vi "CalculatePositionIndex.vi"(8 "error in (no error)":errorcluster, 10 "DragPosition":i32, 11 "OrderSelection in":refnum<class "OrderSelection.lvclass">) -> (0 "error out":errorcluster, 3 "OrderSelection out":refnum<class "OrderSelection.lvclass">)   [LabVIEW 2020, in "OrderSelection.lvclass"]
uses:
  OrderSelection.lvclass
  C:/Program Files/National Instruments/LabVIEW 2020/vi.lib/QSI/QControls/QControl Classes/Picture/Picture.lvclass
  Read ItemGraphic.vi
  Write PositionIndex.vi
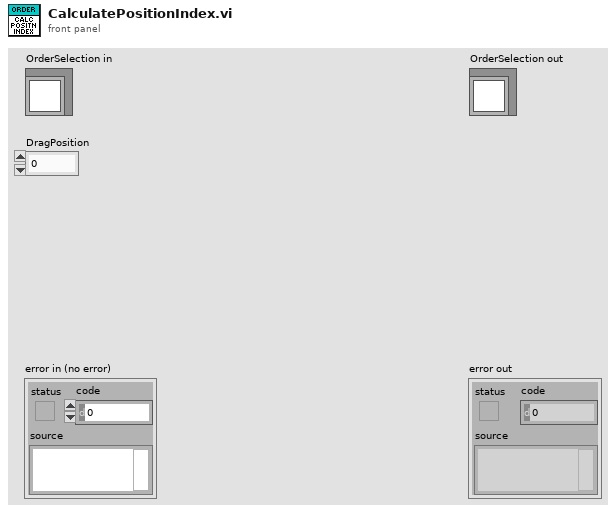
[diagram p1: front panel]
types:
  T1 = typedef "imagedata.ctl" = cluster{"image type":i32, "image depth":i32, "image":u8[], "mask":u8[], "colors":u32[], "Rectangle":cluster{"left":i16, "top":i16, "right":i16, "bottom":i16}}
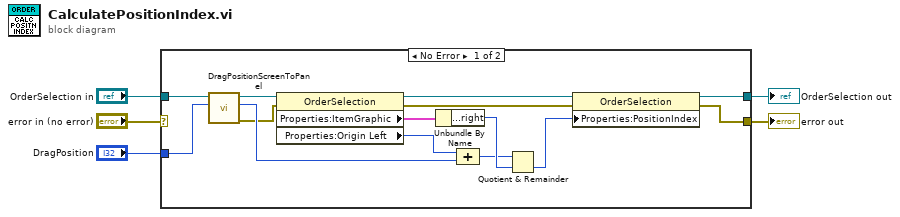
[diagram p0: block diagram]
diagram:
  n1 = case shown="No Error" "error in (no error)" {
    selector: "error in (no error)" -> [_ w21]
    tunnel: [w12 w21] -> w4
    tunnel: [w14 w20] -> w2
    tunnel: "OrderSelection in" -> [w11 w20]
    tunnel: "DragPosition" -> [w9 _]
    frame No Error {
      n2 = call "DragPositionScreenToPanel.vi"("DragPosition (Screen)"=w9, "OrderSelection in"=w11) -> ("error out"=w7:errorcluster, "DragPosition (Panel)"=w8:i32, "OrderSelection out"=w10:refnum<class "OrderSelection.lvclass">)  [unwired: 7 in]
      n3 = property class="OrderSelection"(reference=w10, error in=w7) -> (reference out=w15:refnum<class "OrderSelection.lvclass">, error out=w6:errorcluster, "Properties:ItemGraphic"=w17:T1, "Properties:Origin Left"=w18:i16)
      n4 = Unbundle By Name(w17) -> ("Rectangle.right"=w19:i16)
      n5 = Compound Arithmetic op=ADD(w18, w8) -> (w16:i32)
      n6 = Quotient & Remainder(x=w16, y=w19) -> (floor(x/y)=w13:i32)  [unwired: 1 out]
      n7 = property class="OrderSelection"(reference=w15, error in=w6, "Properties:PositionIndex"=w13) -> (reference out=w14:refnum<class "OrderSelection.lvclass">, error out=w12:errorcluster)
    }
    frame Error {
    }
  }
  "error out" <- w4
  "OrderSelection out" <- w2
